vi "Autonomous Independent.vi"   [LabVIEW 2013]
doc: "This VI is called when autonomous begins, and will automatically be terminated when autonomous ends. You can carry out timed or sensor driven robot movement independently without needing to return to the caller."
uses:
  <vilib>/Rock Robotics/WPI/Solenoid/WPI_SolenoidValue.ctl
  Robot Global Data.vi
  <vilib>/Rock Robotics/WPI/RobotDrive/WPI_RobotDriveGetSetRefNum.vi
  <vilib>/Rock Robotics/WPI/Solenoid/WPI_SolenoidSetEnum.vi
  <vilib>/Rock Robotics/WPI/RobotDrive/WPI_RobotDriveArcadeDrive_Standard(NoSaturation).vi
  <vilib>/Rock Robotics/WPI/Solenoid/Deprecated/WPI_SolenoidGetBool.vi
  <vilib>/Rock Robotics/WPI/Joystick/WPI_JoystickGetSetRefNum.vi
panel:
  # "Be sure to right-click and choose Data Operations>>Make Current Value default if you want to save the array values with the VI"
types:
  T1 = typedef "WPI_JoystickDevRef.ctl" = cluster{"Device":T2}
  T2 = typedef "WPI_JoystickDeviceEnum.ctl" = enum16{"USB 1", "USB 2", "USB 3", "USB 4", "Kinect 1", "Kinect 2"}
  T3 = cluster{"axis 1 (x)":dbl, "axis 2 (y)":dbl, "axis 3 (throttle)":dbl, "axis 4":dbl, "axis 5":dbl, "axis 6":dbl}
  T4 = typedef "WPI_MotorControlDeviceRef.ctl" = cluster{"DeviceStatus":errorcluster, "Type":enum16{"PWM", "CAN"}, "PWM":cluster{"Digital Module":T5, "PWM Channel":T6, "DeadBand":T7}, "CAN":cluster{"Device Number":u8, "Control Mode":T8, "Semaphore":T9, "Max Vout":dbl}, "Invert":bool, "TransformRef":T10, "InvTransformRef":T10}
  T5 = typedef "FPGA_TypedefDigitalModule.ctl" = enum16{"Digital Module 1", "Digital Module 2"}
  T6 = typedef "FPGA_DIOPWMChannel.ctl" = enum8{"PWM 1", "PWM 2", "PWM 3", "PWM 4", "PWM 5", "PWM 6", "PWM 7", "PWM 8", "PWM 9", "PWM 10", "Invalid"}
  T7 = typedef "WPI_PWMDeadband.ctl" = cluster{"Name":string, "maxPositivePwm":i32, "minPositivePwm":i32, "centerPwm":i32, "maxNegativePwm":i32, "minNegativePwm":i32, "angularRange":u16}
  T8 = typedef "WPI_CANJaguar_ControlMode.ctl" = enum8{"Percent VBus", "Current", "Speed", "Position", "Voltage"}
  T9 = typedef "Semaphore RefNum" = refnum<k1>
  T10 = typedef "WPI_PWMTransform_ConPane.ctl" = refnum<vi>
  T11 = typedef "WPI_SolenoidDevRef.ctl" = cluster{"DevStatus":errorcluster, "Solenoid Module":T12, "Forward Solenoid Channel":T13, "Reverse Solenoid Channel":T13}
  T12 = typedef "FPGA_TypedefSolenoidModule.ctl" = enum16{"Solenoid Module 1", "Solenoid Module 2"}
  T13 = typedef "WPI_SolenoidChannel.ctl" = enum8{"Solenoid 1", "Solenoid 2", "Solenoid 3", "Solenoid 4", "Solenoid 5", "Solenoid 6", "Solenoid 7", "Solenoid 8", "Invalid"}
  T14 = typedef "WPI_RobotDriveDevRef.ctl" = cluster{"DevStatus":errorcluster, "Motors[]":T4[], "Square Inputs":bool, "Max Output":dbl, "Isochronous":bool}
  T15 = typedef "WPI_SolenoidValue.ctl" = enum16{"Off", "On", "Forward", "Reverse"}
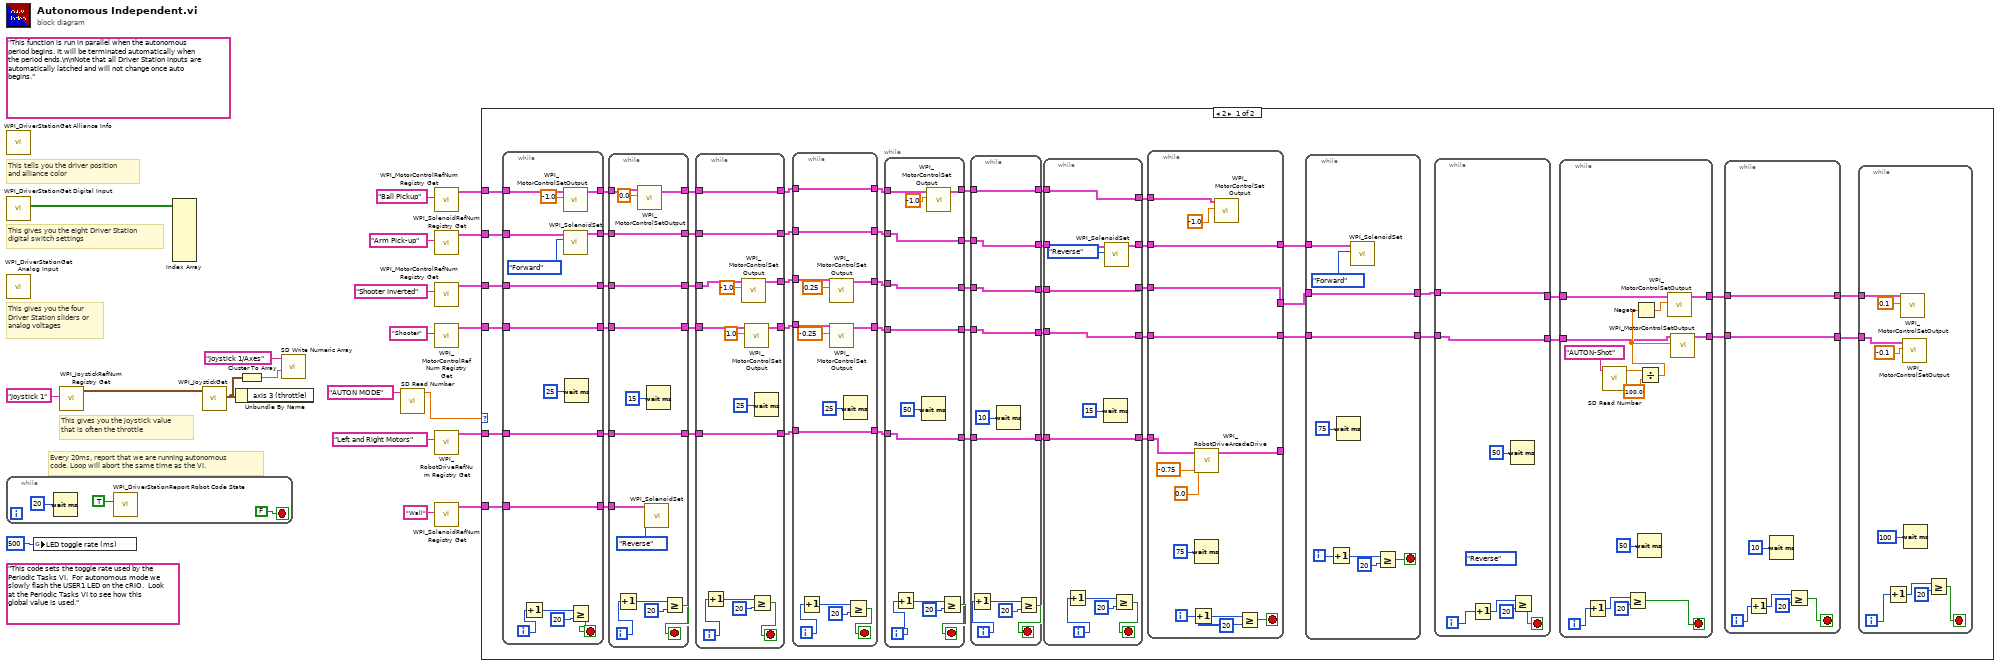
[diagram p0: block diagram]
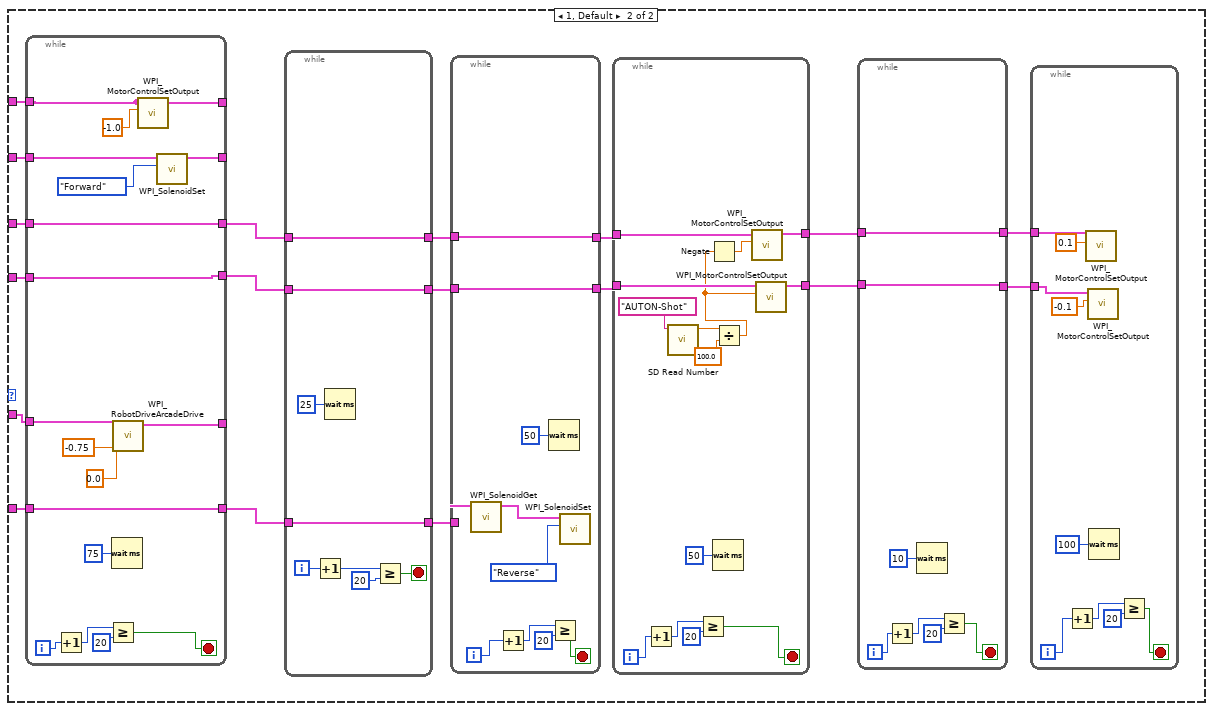
[diagram p2: hidden frame]
diagram:
  (unwired) "This code sets the toggle rate used by the Periodic Tasks VI.  For autonomous mode we slowly flash the USER1 LED on the cRIO.  Look at the Periodic Tasks VI to see how this global value is used."
  (unwired) "This function is run in parallel when the autonomous period begins. It will be terminated automatically when the period ends.\n\nNote that all Driver Station inputs are automatically latched and will not change once auto begins."
  # "Every 20ms, report that we are running autonomous\ncode. Loop will abort the same time as the VI."
  # "This gives you the joystick value\nthat is often the throttle"
  # "This tells you the driver position\nand alliance color"
  # "This gives you the eight Driver Station\ndigital switch settings"
  # "This gives you the four\nDriver Station sliders or\nanalog voltages"
  n1 = call <vilib>:"WPI_DriverStationGet Alliance Info.vi"() -> ()  [unwired: 12 out]
  n2 = call <vilib>:"WPI_DriverStationGet Digital Input.vi"() -> ("Driver Station Digital Input (1-8)"=w21:bool[])  [unwired: 11 out]
  n3 = call <vilib>:"WPI_DriverStationGet Analog Input.vi"() -> ()  [unwired: 12 out]
  n4 = while {
    stop <- FALSE stop-if-true
    n5 = Wait (ms)(milliseconds to wait=u32 20) -> ()  [unwired: 1 out]
    n6 = call <vilib>:"WPI_DriverStationReport Robot Code State.vi"("Autonomous"=TRUE) -> ()  [unwired: 10 in, 1 out]
  }
  n7 = global write "Robot Global Data.vi" "LED toggle rate (ms)"(u32 500 ("LED ms toggle rate")) -> ()
  n8 = call <vilib>:"WPI_JoystickRefNum Registry Get.vi"("refnum name"="Joystick 1") -> ("JoystickDevRef"=w19:T1)  [unwired: 1 in, 9 out]
  n9 = Index Array(array=w21) -> ()  [unwired: 8 in, 8 out]
  n10 = call <vilib>:"WPI_JoystickGet.vi"("JoystickDevRef"=w19) -> ("Axes"=w16:T3)  [unwired: 1 in, 5 out]
  n11 = Unbundle By Name(w16) -> ()  [unwired: 1 out]
  n12 = Cluster To Array(cluster=w16) -> (array=w17:dbl[])
  n13 = call <vilib>:"SD Write Numeric Array.vi"("Numeric Array"=w17, "Name"="Joystick 1/Axes") -> ()  [unwired: 8 in, 2 out]
  n14 = call <vilib>:"SD Read Number.vi"("Name"="AUTON MODE") -> ("Numeric"=w13:dbl)  [unwired: 8 in, 2 out]
  n15 = call <vilib>:"WPI_MotorControlRefNum Registry Get.vi"("refnum name"="Ball Pickup") -> ("MotorControlDevRef"=w1:T4)  [unwired: 9 in, 1 out]
  n16 = call <vilib>:"WPI_SolenoidRefNum Registry Get.vi"("refnum name"="Arm Pick-up") -> ("SolenoidDevRef"=w2:T11)  [unwired: 9 in, 1 out]
  n17 = call <vilib>:"WPI_MotorControlRefNum Registry Get.vi"("refnum name"="Shooter Inverted") -> ("MotorControlDevRef"=w3:T4)  [unwired: 9 in, 1 out]
  n18 = call <vilib>:"WPI_MotorControlRefNum Registry Get.vi"("refnum name"="Shooter") -> ("MotorControlDevRef"=w4:T4)  [unwired: 9 in, 1 out]
  n19 = call <vilib>:"WPI_RobotDriveRefNum Registry Get.vi"("refnum name"="Left and Right Motors") -> ("RobotDriveDevRef"=w6:T14)  [unwired: 9 in, 1 out]
  n20 = call <vilib>:"WPI_SolenoidRefNum Registry Get.vi"("refnum name"="Wall") -> ("SolenoidDevRef"=w5:T11)  [unwired: 9 in, 1 out]
  n21 = case shown="2" w13 {
    tunnel: w6 -> [w69 w246]
    tunnel: w5 -> [w68 w235]
    tunnel: w4 -> [w70 w245]
    tunnel: w3 -> [w71 w244]
    tunnel: w2 -> [w73 w243]
    tunnel: w1 -> [w72 w242]
    frame 2 {
      n22 = while {
        tunnel: w73 -> [w164]
        tunnel: w72 -> [w162]
        tunnel: [w160] -> w64
        tunnel: w71 -> [w160]
        tunnel: w70 -> [w159]
        tunnel: [w159] -> w65
        tunnel: w69 -> [w158]
        tunnel: [w158] -> w66
        tunnel: w68 -> [w157]
        tunnel: [w157] -> w67
        tunnel: [w155] -> w63
        tunnel: [w154] -> w62
        i -> [w165]
        stop <- w166 stop-if-true
        n23 = Increment(x=w165) -> (x+1=w168:i32)
        n24 = call <vilib>:"WPI_MotorControlSetOutput.vi"("Output"=-1.0, "MotorControlDevRef"=w162) -> ("MotorControlDevRef"=w154:T4)  [unwired: 7 in, 2 out]
        n25 = call-poly <vilib>:"WPI_SolenoidSet.vi"("Value"=WPI_SolenoidValue."Forward", "SolenoidDevRef"=w164) -> ("SolenoidDevRef"=w155:T11)  [unwired: 8 in, 1 out]
        n26 = Wait (ms)(milliseconds to wait=u32 25) -> ()  [unwired: 1 out]
        n27 = Greater Or Equal?(x=w168, y=20) -> (x >= y?=w166:bool)
      }
      n28 = while {
        tunnel: w67 -> [w153]
        tunnel: w66 -> [w146]
        tunnel: w65 -> [w145]
        tunnel: w64 -> [w144]
        tunnel: w63 -> [w143]
        tunnel: w62 -> [w142]
        tunnel: [w146] -> w57
        tunnel: [w145] -> w58
        tunnel: [w144] -> w59
        tunnel: [w143] -> w60
        tunnel: [w141] -> w61
        i -> [w148]
        stop <- w149 stop-if-true
        n29 = Increment(x=w148) -> (x+1=w150:i32)
        n30 = call <vilib>:"WPI_MotorControlSetOutput.vi"("Output"=0.0, "MotorControlDevRef"=w142) -> ("MotorControlDevRef"=w141:T4)  [unwired: 7 in, 2 out]
        n31 = call-poly <vilib>:"WPI_SolenoidSet.vi"("Value"=WPI_SolenoidValue."Reverse", "SolenoidDevRef"=w153) -> ()  [unwired: 8 in, 2 out]
        n32 = Wait (ms)(milliseconds to wait=u32 15) -> ()  [unwired: 1 out]
        n33 = Greater Or Equal?(x=w150, y=20) -> (x >= y?=w149:bool)
      }
      n34 = while {
        tunnel: w61 -> [w139]
        tunnel: w60 -> [w138]
        tunnel: w59 -> [w136]
        tunnel: w58 -> [w137]
        tunnel: w57 -> [w133]
        tunnel: [w139] -> w56
        tunnel: [w138] -> w55
        tunnel: [w133] -> w52
        tunnel: [w132] -> w54
        tunnel: [w131] -> w53
        i -> [w127]
        stop <- w128 stop-if-true
        n35 = Increment(x=w127) -> (x+1=w130:i32)
        n36 = call <vilib>:"WPI_MotorControlSetOutput.vi"("Output"=-1.0, "MotorControlDevRef"=w136) -> ("MotorControlDevRef"=w132:T4)  [unwired: 7 in, 2 out]
        n37 = call <vilib>:"WPI_MotorControlSetOutput.vi"("Output"=1.0, "MotorControlDevRef"=w137) -> ("MotorControlDevRef"=w131:T4)  [unwired: 7 in, 2 out]
        n38 = Greater Or Equal?(x=w130, y=20) -> (x >= y?=w128:bool)
        n39 = Wait (ms)(milliseconds to wait=u32 25) -> ()  [unwired: 1 out]
      }
      n40 = while {
        tunnel: w56 -> [w121]
        tunnel: w55 -> [w120]
        tunnel: w54 -> [w124]
        tunnel: w53 -> [w125]
        tunnel: [w121] -> w47
        tunnel: [w120] -> w48
        tunnel: w52 -> [w119]
        tunnel: [w119] -> w51
        tunnel: [w118] -> w50
        tunnel: [w117] -> w49
        i -> [w113]
        stop <- w114 stop-if-true
        n41 = Increment(x=w113) -> (x+1=w115:i32)
        n42 = call <vilib>:"WPI_MotorControlSetOutput.vi"("Output"=-0.25, "MotorControlDevRef"=w125) -> ("MotorControlDevRef"=w118:T4)  [unwired: 7 in, 2 out]
        n43 = call <vilib>:"WPI_MotorControlSetOutput.vi"("Output"=0.25, "MotorControlDevRef"=w124) -> ("MotorControlDevRef"=w117:T4)  [unwired: 7 in, 2 out]
        n44 = Wait (ms)(milliseconds to wait=u32 25) -> ()  [unwired: 1 out]
        n45 = Greater Or Equal?(x=w115, y=20) -> (x >= y?=w114:bool)
      }
      n46 = while {
        tunnel: w51 -> [w104]
        tunnel: w50 -> [w103]
        tunnel: w49 -> [w102]
        tunnel: w48 -> [w101]
        tunnel: w47 -> [w111]
        tunnel: [w104] -> w42
        tunnel: [w103] -> w43
        tunnel: [w102] -> w44
        tunnel: [w101] -> w46
        tunnel: [w100] -> w45
        i -> [w106]
        stop <- w107 stop-if-true
        n47 = Increment(x=w106) -> (x+1=w109:i32)
        n48 = Wait (ms)(milliseconds to wait=u32 50) -> ()  [unwired: 1 out]
        n49 = call <vilib>:"WPI_MotorControlSetOutput.vi"("Output"=-1.0, "MotorControlDevRef"=w111) -> ("MotorControlDevRef"=w100:T4)  [unwired: 7 in, 2 out]
        n50 = Greater Or Equal?(x=w109, y=20) -> (x >= y?=w107:bool)
      }
      n51 = while {
        tunnel: w46 -> [w91]
        tunnel: w45 -> [w90]
        tunnel: w44 -> [w92]
        tunnel: w43 -> [w93]
        tunnel: w42 -> [w94]
        tunnel: [w94] -> w41
        tunnel: [w93] -> w39
        tunnel: [w92] -> w38
        tunnel: [w91] -> w37
        tunnel: [w90] -> w34
        i -> [w96]
        stop <- w95 stop-if-true
        n52 = Increment(x=w96) -> (x+1=w97:i32)
        n53 = Wait (ms)(milliseconds to wait=u32 10) -> ()  [unwired: 1 out]
        n54 = Greater Or Equal?(x=w97, y=20) -> (x >= y?=w95:bool)
      }
      n55 = while {
        tunnel: [w89] -> w40
        tunnel: w41 -> [w89]
        tunnel: w39 -> [w88]
        tunnel: [w88] -> w30
        tunnel: [w87] -> w29
        tunnel: w38 -> [w87]
        tunnel: w37 -> [w81]
        tunnel: [w80] -> w36
        tunnel: [w86] -> w35
        tunnel: w34 -> [w86]
        i -> [w82]
        stop <- w83 stop-if-true
        n56 = Increment(x=w82) -> (x+1=w85:i32)
        n57 = Wait (ms)(milliseconds to wait=u32 15) -> ()  [unwired: 1 out]
        n58 = call-poly <vilib>:"WPI_SolenoidSet.vi"("Value"=WPI_SolenoidValue."Reverse", "SolenoidDevRef"=w81) -> ("SolenoidDevRef"=w80:T11)  [unwired: 8 in, 1 out]
        n59 = Greater Or Equal?(x=w85, y=20) -> (x >= y?=w83:bool)
      }
      n60 = while {
        tunnel: [w223] -> _
        tunnel: w40 -> [w219]
        tunnel: w36 -> [w215]
        tunnel: w35 -> [w218]
        tunnel: [w217] -> w31
        tunnel: w30 -> [w217]
        tunnel: w29 -> [w216]
        tunnel: [w216] -> w28
        tunnel: [w215] -> w25
        i -> [w228]
        stop <- w225 stop-if-true
        n61 = Increment(x=w228) -> (x+1=w227:i32)
        n62 = Wait (ms)(milliseconds to wait=u32 75) -> ()  [unwired: 1 out]
        n63 = call-poly <vilib>:"WPI_RobotDriveArcadeDrive.vi"("Y axis value"=-0.75, "X axis value"=0.0, "RobotDriveDevRef"=w219) -> ("RobotDriveDevRef"=w223:T14)  [unwired: 6 in, 2 out]
        n64 = call <vilib>:"WPI_MotorControlSetOutput.vi"("Output"=-1.0, "MotorControlDevRef"=w218) -> ()  [unwired: 7 in, 3 out]
        n65 = Greater Or Equal?(x=w227, y=20) -> (x >= y?=w225:bool)
      }
      n66 = while {
        tunnel: [w172] -> w32
        tunnel: w31 -> [w172]
        tunnel: w28 -> [w171]
        tunnel: [w171] -> w27
        tunnel: w25 -> [w170]
        i -> [w175]
        stop <- w174 stop-if-true
        n67 = Increment(x=w175) -> (x+1=w176:i32)
        n68 = Wait (ms)(milliseconds to wait=u32 75) -> ()  [unwired: 1 out]
        n69 = call-poly <vilib>:"WPI_SolenoidSet.vi"("Value"=WPI_SolenoidValue."Forward", "SolenoidDevRef"=w170) -> ()  [unwired: 8 in, 2 out]
        n70 = Greater Or Equal?(x=w176, y=20) -> (x >= y?=w174:bool)
      }
      n71 = while {
        tunnel: [w209] -> w33
        tunnel: w32 -> [w209]
        tunnel: w27 -> [w208]
        tunnel: [w208] -> w26
        i -> [w212]
        stop <- w211 stop-if-true
        (unwired) WPI_SolenoidValue."Reverse" ("Value")
        n72 = Increment(x=w212) -> (x+1=w213:i32)
        n73 = Wait (ms)(milliseconds to wait=u32 50) -> ()  [unwired: 1 out]
        n74 = Greater Or Equal?(x=w213, y=20) -> (x >= y?=w211:bool)
      }
      n75 = while {
        tunnel: [w203] -> w77
        tunnel: [w202] -> w76
        tunnel: w33 -> [w195]
        tunnel: w26 -> [w194]
        i -> [w205]
        stop <- w204 stop-if-true
        n76 = Increment(x=w205) -> (x+1=w207:i32)
        n77 = call <vilib>:"SD Read Number.vi"("Name"="AUTON-Shot") -> ("Numeric"=w198:dbl)  [unwired: 8 in, 2 out]
        n78 = Greater Or Equal?(x=w207, y=20) -> (x >= y?=w204:bool)
        n79 = Wait (ms)(milliseconds to wait=u32 50) -> ()  [unwired: 1 out]
        n80 = Divide(x=w198, y=100.0) -> (x/y=w197:dbl)
        n81 = Negate(x=w197) -> (-x=w199:dbl)
        n82 = call <vilib>:"WPI_MotorControlSetOutput.vi"("Output"=w199, "MotorControlDevRef"=w194) -> ("MotorControlDevRef"=w202:T4)  [unwired: 7 in, 2 out]
        n83 = call <vilib>:"WPI_MotorControlSetOutput.vi"("Output"=w197, "MotorControlDevRef"=w195) -> ("MotorControlDevRef"=w203:T4)  [unwired: 7 in, 2 out]
      }
      n84 = while {
        tunnel: w77 -> [w189]
        tunnel: w76 -> [w188]
        tunnel: [w189] -> w74
        tunnel: [w188] -> w75
        i -> [w190]
        stop <- w191 stop-if-true
        n85 = Increment(x=w190) -> (x+1=w192:i32)
        n86 = Wait (ms)(milliseconds to wait=u32 10) -> ()  [unwired: 1 out]
        n87 = Greater Or Equal?(x=w192, y=20) -> (x >= y?=w191:bool)
      }
      n88 = while {
        tunnel: w75 -> [w185]
        tunnel: w74 -> [w186]
        i -> [w180]
        stop <- w179 stop-if-true
        n89 = Increment(x=w180) -> (x+1=w182:i32)
        n90 = call <vilib>:"WPI_MotorControlSetOutput.vi"("Output"=0.1, "MotorControlDevRef"=w185) -> ()  [unwired: 7 in, 3 out]
        n91 = call <vilib>:"WPI_MotorControlSetOutput.vi"("Output"=-0.1, "MotorControlDevRef"=w186) -> ()  [unwired: 7 in, 3 out]
        n92 = Wait (ms)(milliseconds to wait=u32 100) -> ()  [unwired: 1 out]
        n93 = Greater Or Equal?(x=w182, y=20) -> (x >= y?=w179:bool)
      }
    }
    frame 1, Default {
      n94 = while {
        tunnel: w246 -> [w306]
        tunnel: [w304] -> _
        tunnel: [w303] -> w232
        tunnel: w245 -> [w303]
        tunnel: w244 -> [w302]
        tunnel: [w302] -> w229
        tunnel: w243 -> [w297]
        tunnel: w242 -> [w296]
        tunnel: [w296] -> _
        tunnel: [w297] -> _
        tunnel: [w299] -> w234
        tunnel: w235 -> [w299]
        i -> [w310]
        stop <- w307 stop-if-true
        n95 = Increment(x=w310) -> (x+1=w309:i32)
        n96 = Greater Or Equal?(x=w309, y=20) -> (x >= y?=w307:bool)
        n97 = Wait (ms)(milliseconds to wait=u32 75) -> ()  [unwired: 1 out]
        n98 = call-poly <vilib>:"WPI_RobotDriveArcadeDrive.vi"("Y axis value"=-0.75, "X axis value"=0.0, "RobotDriveDevRef"=w306) -> ("RobotDriveDevRef"=w304:T14)  [unwired: 6 in, 2 out]
        n99 = call <vilib>:"WPI_MotorControlSetOutput.vi"("Output"=-1.0, "MotorControlDevRef"=w296) -> ()  [unwired: 7 in, 3 out]
        n100 = call-poly <vilib>:"WPI_SolenoidSet.vi"("Value"=WPI_SolenoidValue."Forward", "SolenoidDevRef"=w297) -> ()  [unwired: 8 in, 2 out]
      }
      n101 = while {
        tunnel: w234 -> [w254]
        tunnel: [w254] -> w233
        tunnel: w232 -> [w253]
        tunnel: [w253] -> w231
        tunnel: [w252] -> w230
        tunnel: w229 -> [w252]
        i -> [w249]
        stop <- w248 stop-if-true
        n102 = Increment(x=w249) -> (x+1=w250:i32)
        n103 = Wait (ms)(milliseconds to wait=u32 25) -> ()  [unwired: 1 out]
        n104 = Greater Or Equal?(x=w250, y=20) -> (x >= y?=w248:bool)
      }
      n105 = while {
        tunnel: w231 -> [w289]
        tunnel: w230 -> [w290]
        tunnel: [w290] -> w241
        tunnel: [w289] -> w240
        tunnel: w233 -> [w287]
        i -> [w292]
        stop <- w291 stop-if-true
        n106 = call-poly <vilib>:"WPI_SolenoidGet.vi"("SolenoidDevRef"=w287) -> ("SolenoidDevRef"=w285:T11)  [unwired: 8 in, 2 out]
        n107 = Increment(x=w292) -> (x+1=w293:i32)
        n108 = Wait (ms)(milliseconds to wait=u32 50) -> ()  [unwired: 1 out]
        n109 = Greater Or Equal?(x=w293, y=20) -> (x >= y?=w291:bool)
        n110 = call-poly <vilib>:"WPI_SolenoidSet.vi"("Value"=WPI_SolenoidValue."Reverse", "SolenoidDevRef"=w285) -> ()  [unwired: 8 in, 2 out]
      }
      n111 = while {
        tunnel: w241 -> [w280]
        tunnel: w240 -> [w279]
        tunnel: [w278] -> w239
        tunnel: [w277] -> w238
        i -> [w282]
        stop <- w281 stop-if-true
        n112 = Increment(x=w282) -> (x+1=w284:i32)
        n113 = call <vilib>:"SD Read Number.vi"("Name"="AUTON-Shot") -> ("Numeric"=w273:dbl)  [unwired: 8 in, 2 out]
        n114 = Greater Or Equal?(x=w284, y=20) -> (x >= y?=w281:bool)
        n115 = Wait (ms)(milliseconds to wait=u32 50) -> ()  [unwired: 1 out]
        n116 = Divide(x=w273, y=100.0) -> (x/y=w272:dbl)
        n117 = Negate(x=w272) -> (-x=w274:dbl)
        n118 = call <vilib>:"WPI_MotorControlSetOutput.vi"("Output"=w274, "MotorControlDevRef"=w280) -> ("MotorControlDevRef"=w277:T4)  [unwired: 7 in, 2 out]
        n119 = call <vilib>:"WPI_MotorControlSetOutput.vi"("Output"=w272, "MotorControlDevRef"=w279) -> ("MotorControlDevRef"=w278:T4)  [unwired: 7 in, 2 out]
      }
      n120 = while {
        tunnel: w239 -> [w266]
        tunnel: w238 -> [w265]
        tunnel: [w266] -> w236
        tunnel: [w265] -> w237
        i -> [w267]
        stop <- w268 stop-if-true
        n121 = Increment(x=w267) -> (x+1=w269:i32)
        n122 = Wait (ms)(milliseconds to wait=u32 10) -> ()  [unwired: 1 out]
        n123 = Greater Or Equal?(x=w269, y=20) -> (x >= y?=w268:bool)
      }
      n124 = while {
        tunnel: w237 -> [w262]
        tunnel: w236 -> [w263]
        i -> [w257]
        stop <- w256 stop-if-true
        n125 = Increment(x=w257) -> (x+1=w259:i32)
        n126 = call <vilib>:"WPI_MotorControlSetOutput.vi"("Output"=0.1, "MotorControlDevRef"=w262) -> ()  [unwired: 7 in, 3 out]
        n127 = call <vilib>:"WPI_MotorControlSetOutput.vi"("Output"=-0.1, "MotorControlDevRef"=w263) -> ()  [unwired: 7 in, 3 out]
        n128 = Wait (ms)(milliseconds to wait=u32 100) -> ()  [unwired: 1 out]
        n129 = Greater Or Equal?(x=w259, y=20) -> (x >= y?=w256:bool)
      }
    }
  }
